vi "Resistance_to_Temp_Conversion(SubVI).vi"(11 "Scalar":dbl) -> (3 "Result":dbl)   [LabVIEW 2013]
uses:
  <vilib>/express/express arith-compare/Formula/XNode/ExpressFormulaBlockNode.xnode
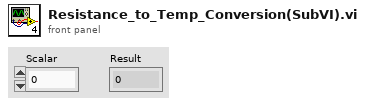
[diagram p1: front panel]
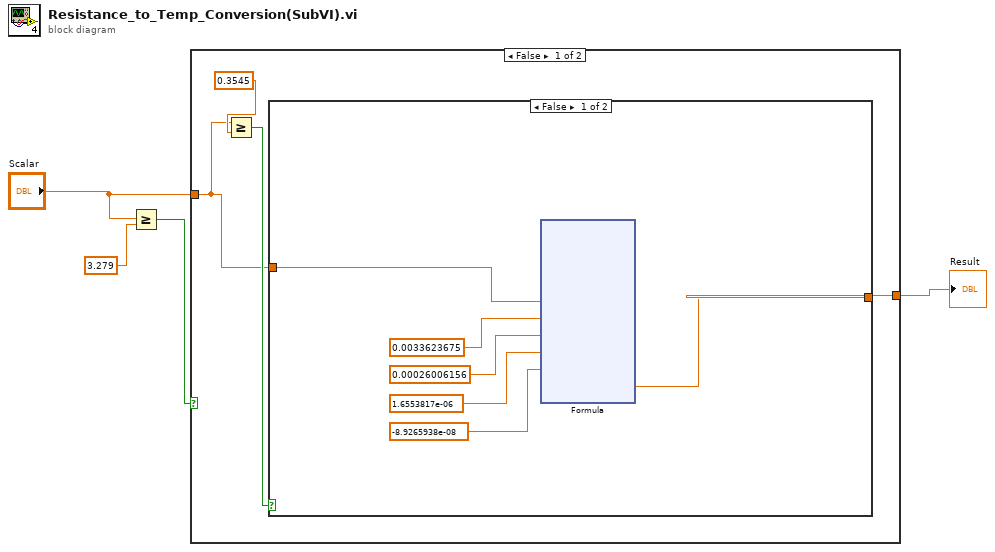
[diagram p0: block diagram]
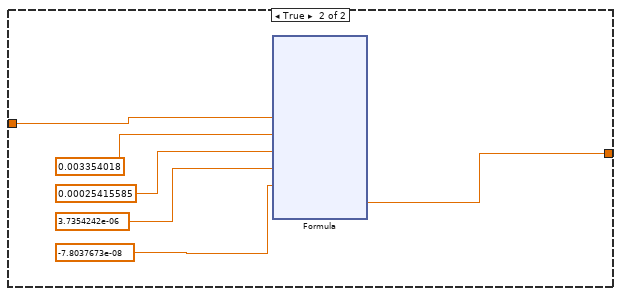
[diagram p2: hidden frame]
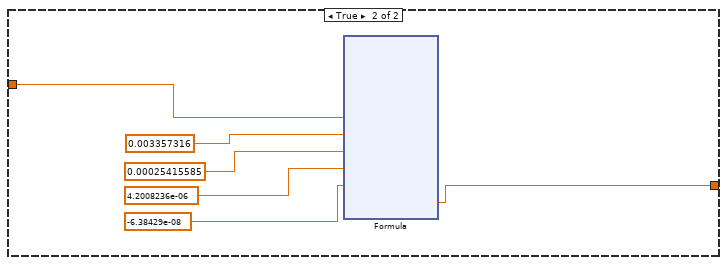
[diagram p3: hidden frame]
diagram:
  n1 = Greater Or Equal?(x="Scalar", y=3.279) -> (x >= y?=w1:bool)
  n2 = case shown="False" w1 {
    tunnel: "Scalar" -> [w5 w58]
    tunnel: [w8 w53] -> w2
    frame False {
      n3 = Greater Or Equal?(x=w5, y=0.3545) -> (x >= y?=w7:bool)
      n4 = case shown="False" w7 {
        tunnel: w5 -> [w14 w36]
        tunnel: [w13 w32] -> w8
        frame False {
          n5 = xnode "Formula"("Ratio"=w14, "a"=0.0033623675, "b"=0.00026006156, "c"=1.6553817e-06, "d"=-8.9265938e-08) -> ("Result"=w13:dbl)  [unwired: 1 in, 1 out]
        }
        frame True {
          n6 = xnode "Formula"("Ratio"=w36, "a"=0.003354018, "b"=0.00025415585, "c"=3.7354242e-06, "d"=-7.8037673e-08) -> ("Result"=w32:dbl)  [unwired: 1 in, 1 out]
        }
      }
    }
    frame True {
      n7 = xnode "Formula"("Ratio"=w58, "a"=0.003357316, "b"=0.00025415585, "c"=4.2008236e-06, "d"=-6.38429e-08) -> ("Result"=w53:dbl)  [unwired: 1 in, 1 out]
    }
  }
  "Result" <- w2
